vi "Set Image Type.vi"(8 "error in (no error)":errorcluster, 10 "Image Type(U8)":T1 items=["Grayscale (U8)", "Grayscale (I16)", "Grayscale (SGL)", "Complex (CSG)", "RGB (U32)", "HSL (U32)", "RGB (U64)", "Grayscale (U16)"], 11 "ImageOperation in":refnum<class "ImageOperation.lvclass">) -> (0 "error out":errorcluster, 3 "ImageOperation out":refnum<class "ImageOperation.lvclass">)   [LabVIEW 2015, in "ImageOperation.lvclass"]
uses:
  ImageOperation.lvclass
  ImageOperation.lvclass/ImageOperation.ctl
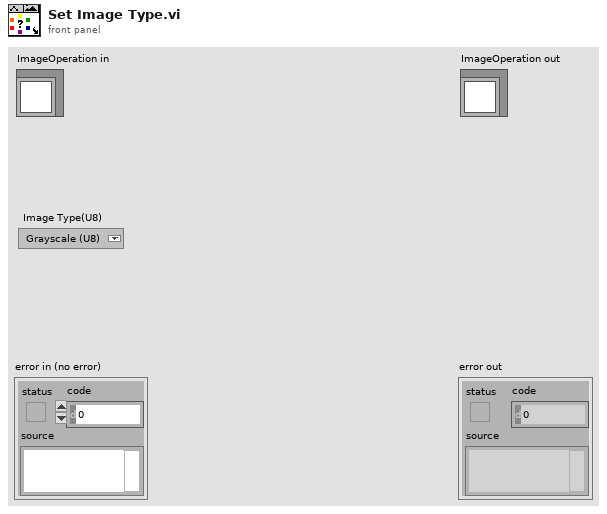
[diagram p1: front panel]
types:
  T1 = typedef "Image Type" = u32
  T2 = typedef "IMAQ Image.ctl" = refnum<image>
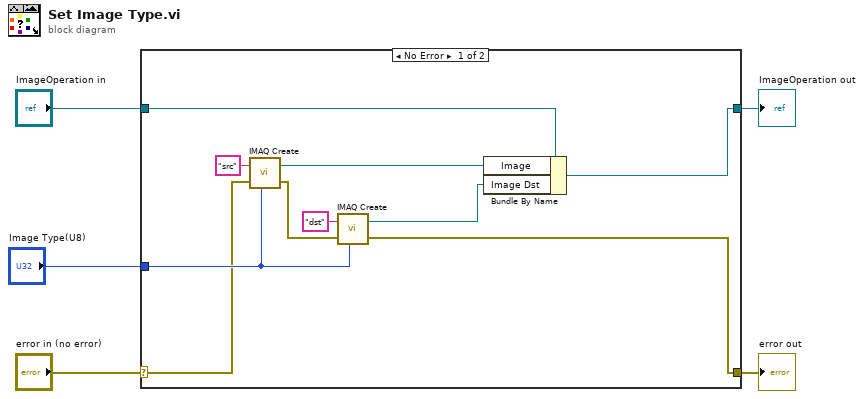
[diagram p0: block diagram]
diagram:
  n1 = case shown="No Error" "error in (no error)" {
    selector: "error in (no error)" -> [w12 w17]
    tunnel: [w6 w17] -> w4
    tunnel: [w7 w16] -> w2
    tunnel: "ImageOperation in" -> [w10 w16]
    tunnel: "Image Type(U8)" -> [w13 _]
    frame No Error {
      n2 = call "IMAQ Create"("Image Name"="src", "Image Type"=w13, "error in (no error)"=w12) -> ("New Image"=w9:T2, "error out"=w11:errorcluster)  [unwired: 2 in]
      n3 = call "IMAQ Create"("Image Name"="dst", "Image Type"=w13, "error in (no error)"=w11) -> ("New Image"=w8:T2, "error out"=w6:errorcluster)  [unwired: 2 in]
      n4 = Bundle By Name(cluster=w10, "Image"=w9, "Image Dst"=w8) -> (w7:refnum<class "ImageOperation.lvclass">)
    }
    frame Error {
    }
  }
  "error out" <- w4
  "ImageOperation out" <- w2
